vi "bool to string (sub-vi).vi"(1 "Boolean":bool) -> (0 "String":string)   [LabVIEW 2021]
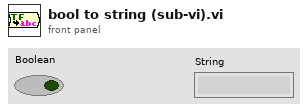
[diagram p1: front panel]
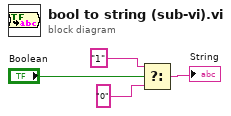
[diagram p0: block diagram]
diagram:
  n1 = Select(t="1", s="Boolean", f="0") -> (s? t:f=→"String":string)
